vi "instrumentProperties_channel_gainLevels.vi"(8 "error in (no error)":errorcluster, 11 "OSAchannel in":refnum<class "OSAchannel.lvclass">) -> (0 "error out":errorcluster, 2 "gainLevels relative":dbl[](array[numeric]), 3 "OSAchannel out":refnum<class "OSAchannel.lvclass">)   [LabVIEW 2010, in "OSAchannel.lvclass"]
uses:
  OSAchannel.lvclass
  OSA20X_misc.lvlib
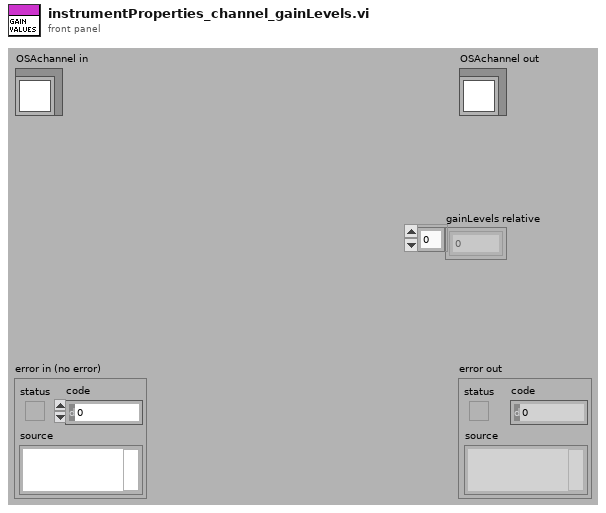
[diagram p1: front panel]
types:
  T1 = typedef "OSA.lvclass/interferogram_smoothing.ctl" = enum16{"NONE", "BINOMIAL", "SAVITSKY_GOLAY", "FOURIER", "MOVING_AVERAGE", "GAUSSIAN"}
  T2 = cluster{"waveMin (cm-1)":sgl, "waveMax (cm-1)":sgl, "gainOffset_auto":bool, "gain":i32, "gain levels nr":u16, "offset":i32, "offset max":u16, "damper available":bool, "damper active":bool, "amplifier type":i32, "detector type":i32, "channelIdx global":u16, "spectrIdx":u16, "waveMeter on":bool, "ref gainLevels rel.":refnum<data-value>, "intfgrm_smooth_width":u16, "intfgrm_smooth_nrOfPasses":u16, "intfgrm_smooth":T1}
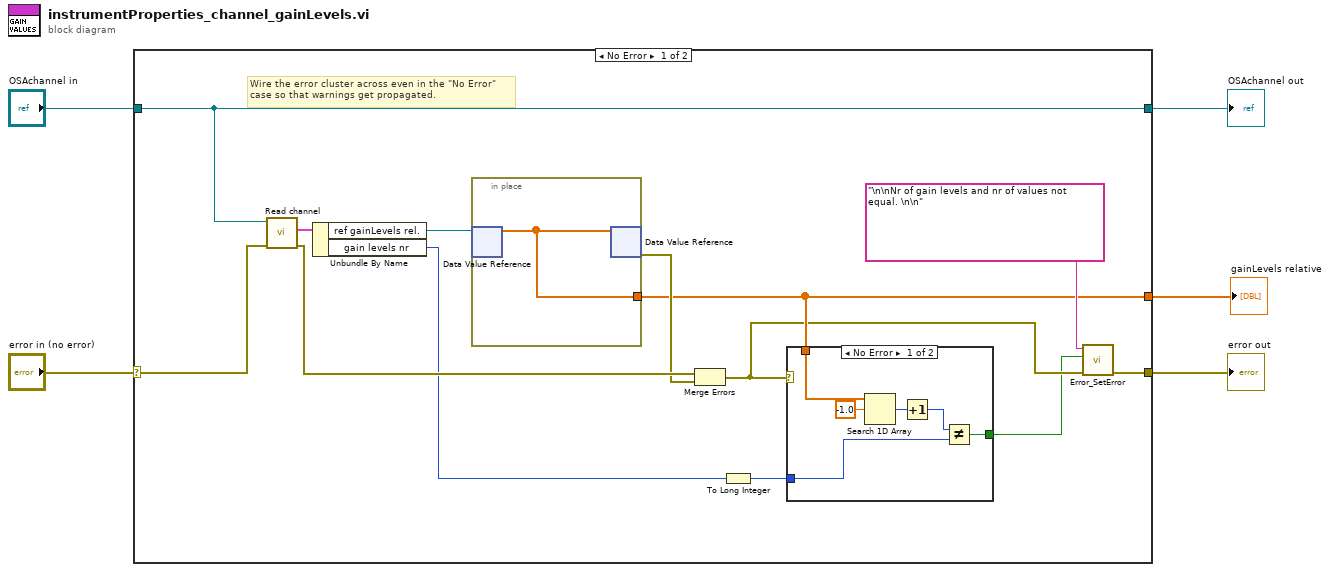
[diagram p0: block diagram]
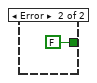
[diagram p2: hidden frame]
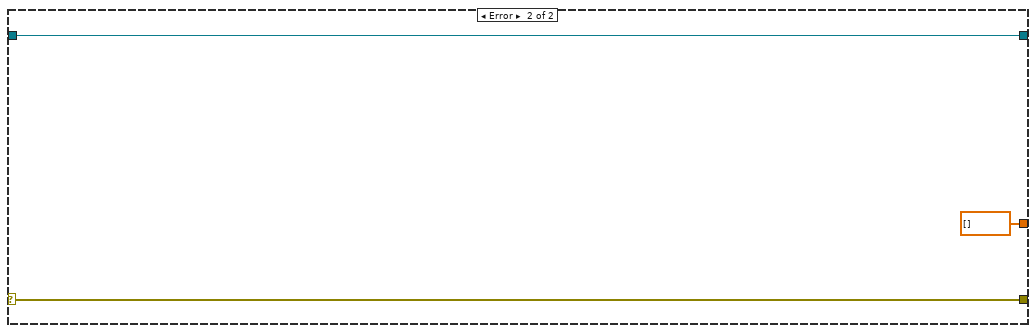
[diagram p3: hidden frame]
diagram:
  n1 = case shown="No Error" "error in (no error)" {
    selector: "error in (no error)" -> [w18 w29]
    tunnel: [w6 w29] -> w4
    tunnel: [w17 w28] -> w2
    tunnel: "OSAchannel in" -> [w17 w28]
    tunnel: [w9 dbl[] []] -> w1
    frame No Error {
      # "Wire the error cluster across even in the \"No Error\"\ncase so that warnings get propagated."
      n2 = call "Read channel.vi"("error in (no error)"=w18, "OSAchannel in"=w17) -> ("error out"=w14:errorcluster, "channel"=w16:T2)  [unwired: 7 in, 1 out]
      n3 = Unbundle By Name(w16) -> ("ref gainLevels rel."=w15:refnum<data-value>, "gain levels nr"=w11:u16)
      n4 = in-place {
        in-place-border: [w26] -> w9
        n5 = in-place-dvr #1(w15) -> (w26:dbl[])  [unwired: 1 out]
        n6 = in-place-dvr #1(w26) -> (w13:errorcluster)  [unwired: 1 out]
      }
      n7 = Merge Errors(w14, w13) -> (w8:errorcluster)
      n8 = To Long Integer(number=w11) -> (32bit integer=w10:i32)
      n9 = case shown="No Error" w8 {
        tunnel: w9 -> [w21 _]
        tunnel: w10 -> [w23 _]
        tunnel: [w20 FALSE] -> w7
        frame No Error {
          n10 = Search 1D Array(1D array=w21, element=-1.0) -> (index of element=w24:i32)  [unwired: 1 in]
          n11 = Increment(x=w24) -> (x+1=w22:i32)
          n12 = Not Equal?(x=w22, y=w23) -> (x != y?=w20:bool)
        }
        frame Error {
        }
      }
      n13 = call "Error_SetError.vi"("error in"=w8, "status (true)"=w7, "source(\"\")"="\n\nNr of gain levels and nr of values not equal. \n\n" ("source(\"\")")) -> ("error out"=w6:errorcluster)  [unwired: 4 in]
    }
    frame Error {
    }
  }
  "error out" <- w4
  "OSAchannel out" <- w2
  "gainLevels relative" <- w1
